vi "ElevFF_MaxAchieveVelocity.vi"(9 "Acceleration":dbl, 10 "MaxVoltage":dbl, 11 "in ELEV_FF":T1 {"Kg" format="%13.5p"; "Ka" format="%13.5p"; "Kv" format="%13.5p"; "Ks" format="%13.5p"}) -> (3 "MaxVelocity":dbl)   [LabVIEW 2019, in "Trajectory_Library.lvlib"]
doc: "Calculates the maximum achievable velocity given a maximum voltage supply and an acceleration. Useful for ensuring that velocity and acceleration constraints for a trapezoidal profile are simultaneously achievable - enter the acceleration constraint, and this will give you a simultaneously-achievable velocity constraint.\n \nInputs: \n - ElevFF -- The ElevFF data cluster\n - maxVoltage -- The maximum voltage that can be supplied to the elevator.\n - acceleration -- The acceleration of the elevator.\n\nOutputs:\n - MaxVelocity -- The maximum possible velocity at the given acceleration."
uses:
  Trajectory_Library.lvlib
  TypeDef/ELEV_FF.ctl
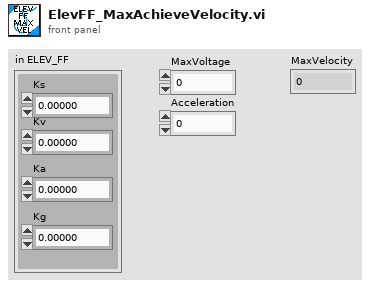
[diagram p1: front panel]
types:
  T1 = typedef "Trajectory_Library.lvlib/ELEV_FF.ctl" = cluster{"Ks":dbl, "Kv":dbl, "Ka":dbl, "Kg":dbl}
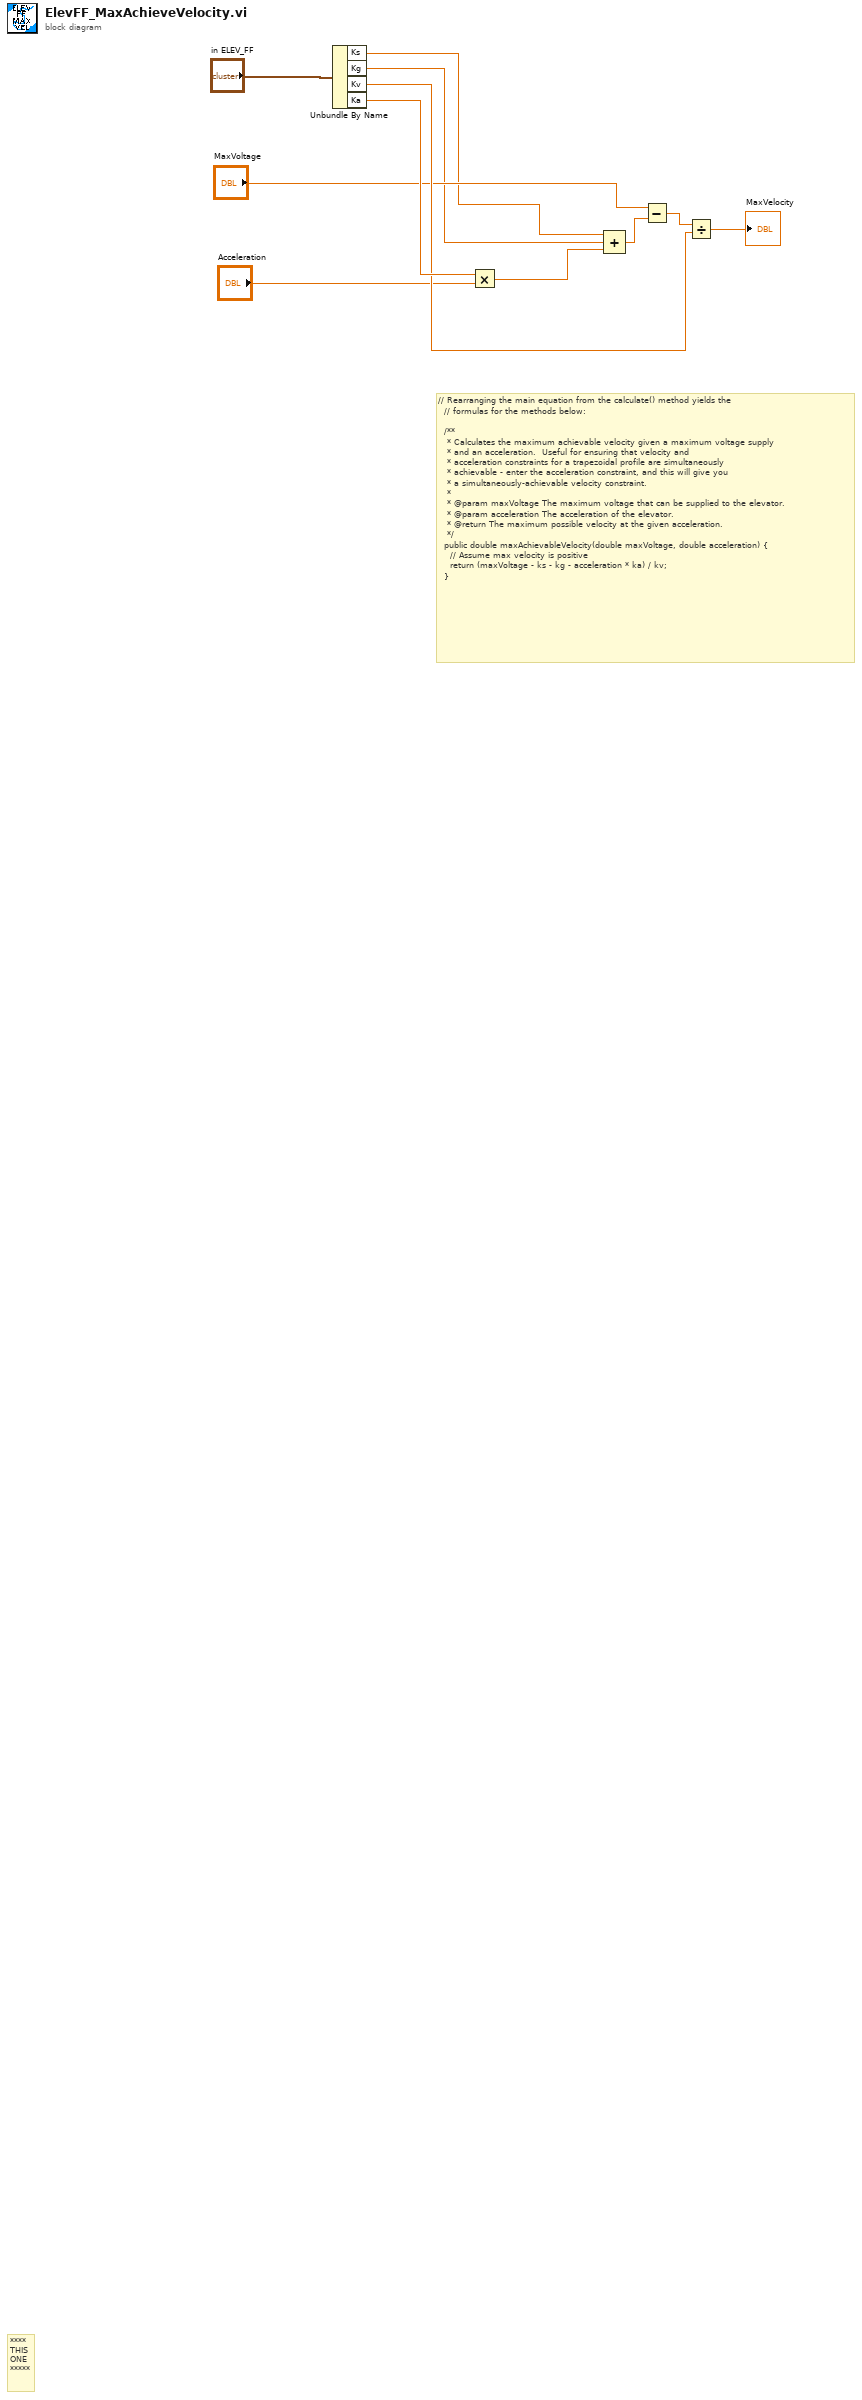
[diagram p0: block diagram]
diagram:
  # "// Rearranging the main equation from the calculate() method yields the\n  // formulas for the methods below:\n\n  /**\n   * Calculates the maximum achievable velocity given a maximum voltage supply\n   * and an acceleration.  Useful for ensuring that velocity and\n   * acceleration constraints for a trapezoidal profile are simultaneously\n   * achievable - enter the acceleration constraint, and this will give you\n   * a simultaneously-achievable velocity constraint.\n   *\n   * @param maxVoltage The maximum voltage that can be supplied to the elevator.\n   * @param acceleration The acceleration of the elevator.\n   * @return The maximum possible velocity at the given acceleration.\n   */\n  public double maxAchievableVelocity(double maxVoltage, double acceleration) {\n    // Assume max velocity is positive\n    return (maxVoltage - ks - kg - acceleration * ka) / kv;\n  }"
  # "****\nTHIS\nONE\n*****"
  n1 = Unbundle By Name("in ELEV_FF") -> ("Ks"=w4:dbl, "Kg"=w2:dbl, "Kv"=w8:dbl, "Ka"=w10:dbl)
  n2 = Multiply(x=w10, y="Acceleration") -> (x*y=w3:dbl)
  n3 = Compound Arithmetic op=ADD(w4, w2, w3) -> (w6:dbl)
  n4 = Subtract(x="MaxVoltage", y=w6) -> (x-y=w7:dbl)
  n5 = Divide(x=w7, y=w8) -> (x/y=→"MaxVelocity":dbl)
